vi "DeleteAll.vi"(8 "error in (no error)":errorcluster, 11 "Refnum in":T1) -> (0 "error out":errorcluster, 3 "Refnum out":T1)   [LabVIEW 2018]
uses:
  <vilib>/httpClient/ClientHandle.ctl
  <vilib>/httpClient/LabVIEWHTTPClient.lvlib
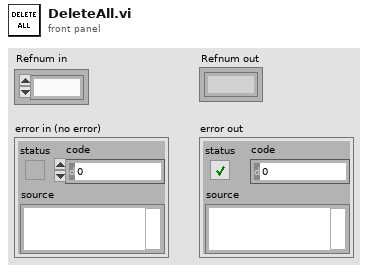
[diagram p1: front panel]
types:
  T1 = typedef "LabVIEWHTTPClient.lvlib/ClientHandle.ctl" = refnum<k1>
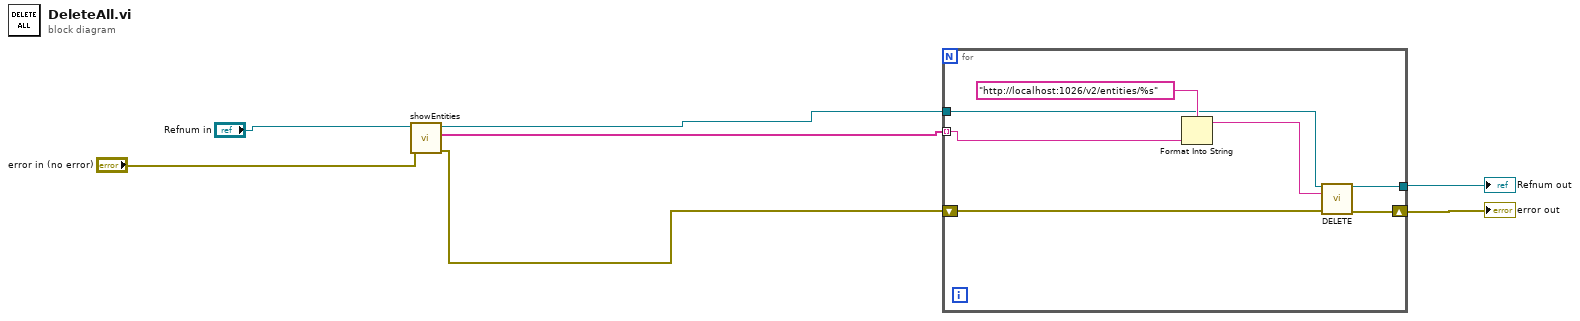
[diagram p0: block diagram]
diagram:
  n1 = call "showEntities.vi"("error in (no error)"="error in (no error)", "Refnum in"="Refnum in") -> ("error out"=w4:errorcluster, "EntitiesList"=w2:string[], "Refnum out"=w3:T1)  [unwired: 7 in]
  n2 = for {
    tunnel: w2 -> [w12] mode=indexing
    tunnel: w3 -> [w11]
    shift-right: [w9] -> w6
    shift-left: w4 -> [w10]
    tunnel: [w8] -> w5
    n3 = Format Into String(format string="http://localhost:1026/v2/entities/%s", w12) -> (resulting string=w13:string)  [unwired: 2 in, 1 out]
    n4 = call <vilib>:"DELETE.vi"("client handle"=w11, "url"=w13, "error in (no error)"=w10) -> ("client handle out"=w8:T1, "error out"=w9:errorcluster)  [unwired: 9 in, 2 out]
  }
  "Refnum out" <- w5
  "error out" <- w6
